vi "绝对码变相对码.vi"(1 "输入信息代码":u32[](array[numeric])) -> (0 "相对码":i32[](array[numeric]))   [LabVIEW 2013]
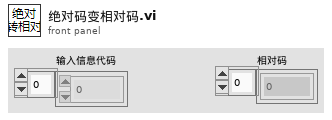
[diagram p1: front panel]
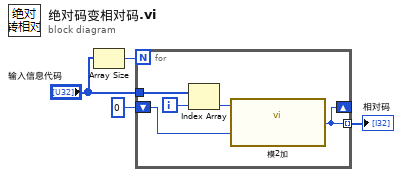
[diagram p0: block diagram]
diagram:
  n1 = Array Size(array="输入信息代码") -> (size(s)=w4:i32)
  n2 = for {
    N: w4 -> [_]
    tunnel: "输入信息代码" -> [w9]
    shift-right: [w5] -> _
    shift-left: 0 -> [w6]
    tunnel: [w5] -> w1 mode=indexing
    i -> [w8]
    n3 = Index Array(array=w9, index=w8) -> (element=w7:u32)
    n4 = call "模2加.vi"("b"=w6, "a"=w7) -> ("c"=w5:u32)
  }
  "相对码" <- w1
